vi "Filter Axis Spikes.vi"(8 "Error In":errorcluster, 9 "Axis Enum":T1=enum."Z-axis", 11 "Current Reading":dbl) -> (0 "Error Out":errorcluster, 1 "Axis Enum out":T1=enum."Z-axis", 3 "Filtered Reading":dbl, 5 "Peak Detected?":bool)   [LabVIEW 2013]
doc: "This sub-VI detects peaks due to noise in the positions read by axis encoders and replaces these peaks with\nthe previous value of the axis position."
uses:
  Controls/table_axis_enum.ctl
  <vilib>/ptbypt/NI_PtbyPt.lvlib
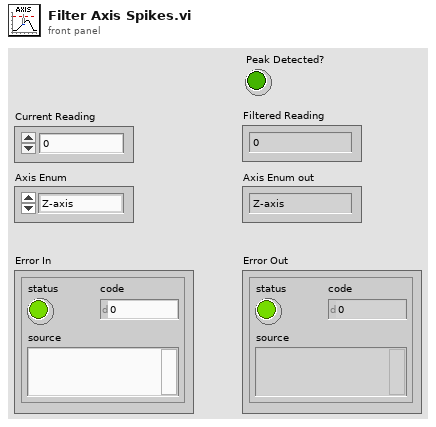
[diagram p1: front panel]
types:
  T1 = typedef "table_axis_enum.ctl" = enum16{"X-axis", "Y-axis", "Z-axis", "W-axis"}
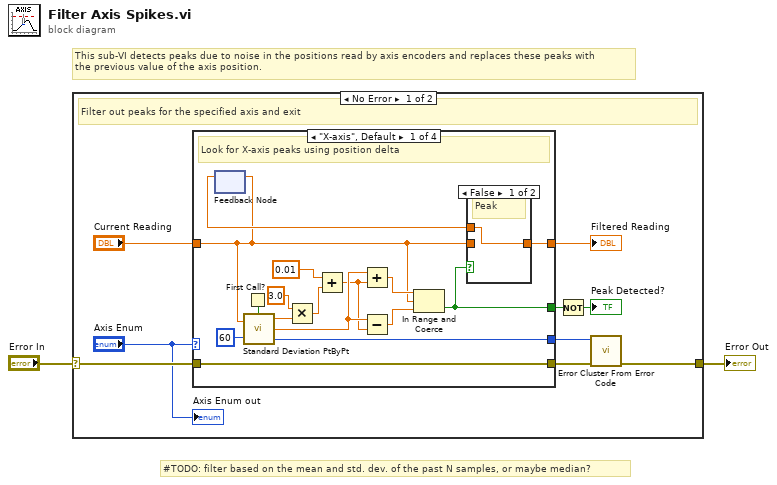
[diagram p0: block diagram]
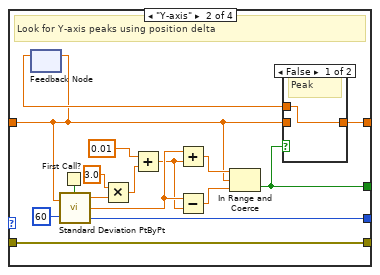
[diagram p3: hidden frame]
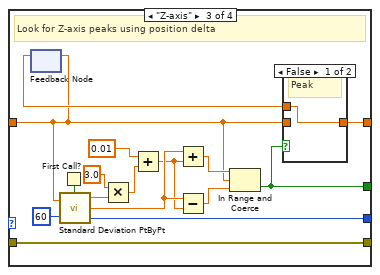
[diagram p5: hidden frame]
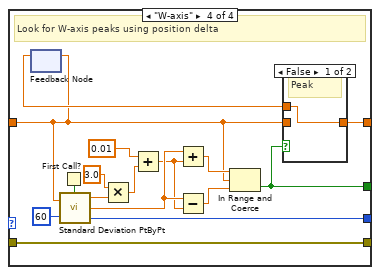
[diagram p7: hidden frame]
diagram:
  # "#TODO: filter based on the mean and std. dev. of the past N samples, or maybe median?"
  # "This sub-VI detects peaks due to noise in the positions read by axis encoders and replaces these peaks with\nthe previous value of the axis position."
  n1 = case shown="No Error" "Error In" {
    selector: "Error In" -> [w11 w84]
    tunnel: [w5 w84] -> w1
    frame No Error {
      # "Filter out peaks for the specified axis and exit"
      n2 = case shown="\"X-axis\", Default" "Axis Enum" {
        tunnel: w11 -> [w27 w45 w63 w81]
        tunnel: [w27 w45 w63 w81] -> w6
        tunnel: "Current Reading" -> [w15 w33 w51 w69]
        tunnel: [w16 w34 w52 w70] -> w9
        tunnel: [w20 w38 w56 w74] -> w8
        tunnel: [w22 w40 w58 w76] -> w4
        frame "X-axis", Default {
          # "Look for X-axis peaks using position delta"
          n3 = feedback-in #1(w15) -> ()
          n4 = feedback #1() -> (w21:dbl)  [unwired: 1 in]
          n5 = First Call?() -> (First Call?: T/F=w26:bool)
          n6 = call <vilib>:"Standard Deviation PtByPt.vi"("x"=w15, "sample length"=60, "initialize"=w26) -> ("standard deviation"=w24:dbl, "mean"=w17:dbl, "error"=w22:i32)
          n7 = Multiply(x=3.0, y=w24) -> (x*y=w14:dbl)
          n8 = Add(x=0.01, y=w14) -> (x+y=w13:dbl)
          n9 = Add(x=w17, y=w13) -> (x+y=w18:dbl)
          n10 = Subtract(x=w17, y=w13) -> (x-y=w19:dbl)
          n11 = In Range and Coerce(upper limit=w18, x=w15, lower limit=w19) -> (In Range?=w16:bool)  [unwired: 1 out]
          n12 = case shown="False" w16 {
            tunnel: w15 -> [_ w29]
            tunnel: w21 -> [w28 _]
            tunnel: [w28 w29] -> w20
            frame False {
              # "Peak"
            }
            frame True {
              # "No peak"
            }
          }
        }
        frame "Y-axis" {
          # "Look for Y-axis peaks using position delta"
          n13 = feedback-in #2(w33) -> ()
          n14 = feedback #2() -> (w39:dbl)  [unwired: 1 in]
          n15 = First Call?() -> (First Call?: T/F=w44:bool)
          n16 = call <vilib>:"Standard Deviation PtByPt.vi"("x"=w33, "sample length"=60, "initialize"=w44) -> ("standard deviation"=w42:dbl, "mean"=w35:dbl, "error"=w40:i32)
          n17 = Multiply(x=3.0, y=w42) -> (x*y=w32:dbl)
          n18 = Add(x=0.01, y=w32) -> (x+y=w31:dbl)
          n19 = Add(x=w35, y=w31) -> (x+y=w36:dbl)
          n20 = Subtract(x=w35, y=w31) -> (x-y=w37:dbl)
          n21 = In Range and Coerce(upper limit=w36, x=w33, lower limit=w37) -> (In Range?=w34:bool)  [unwired: 1 out]
          n22 = case shown="False" w34 {
            tunnel: w33 -> [_ w47]
            tunnel: w39 -> [w46 _]
            tunnel: [w46 w47] -> w38
            frame False {
              # "Peak"
            }
            frame True {
              # "No peak"
            }
          }
        }
        frame "Z-axis" {
          # "Look for Z-axis peaks using position delta"
          n23 = feedback-in #3(w51) -> ()
          n24 = feedback #3() -> (w57:dbl)  [unwired: 1 in]
          n25 = First Call?() -> (First Call?: T/F=w62:bool)
          n26 = call <vilib>:"Standard Deviation PtByPt.vi"("x"=w51, "sample length"=60, "initialize"=w62) -> ("standard deviation"=w60:dbl, "mean"=w53:dbl, "error"=w58:i32)
          n27 = Multiply(x=3.0, y=w60) -> (x*y=w50:dbl)
          n28 = Add(x=0.01, y=w50) -> (x+y=w49:dbl)
          n29 = Add(x=w53, y=w49) -> (x+y=w54:dbl)
          n30 = Subtract(x=w53, y=w49) -> (x-y=w55:dbl)
          n31 = In Range and Coerce(upper limit=w54, x=w51, lower limit=w55) -> (In Range?=w52:bool)  [unwired: 1 out]
          n32 = case shown="False" w52 {
            tunnel: w51 -> [_ w65]
            tunnel: w57 -> [w64 _]
            tunnel: [w64 w65] -> w56
            frame False {
              # "Peak"
            }
            frame True {
              # "No peak"
            }
          }
        }
        frame "W-axis" {
          # "Look for W-axis peaks using position delta"
          n33 = feedback-in #4(w69) -> ()
          n34 = feedback #4() -> (w75:dbl)  [unwired: 1 in]
          n35 = First Call?() -> (First Call?: T/F=w80:bool)
          n36 = call <vilib>:"Standard Deviation PtByPt.vi"("x"=w69, "sample length"=60, "initialize"=w80) -> ("standard deviation"=w78:dbl, "mean"=w71:dbl, "error"=w76:i32)
          n37 = Multiply(x=3.0, y=w78) -> (x*y=w68:dbl)
          n38 = Add(x=0.01, y=w68) -> (x+y=w67:dbl)
          n39 = Add(x=w71, y=w67) -> (x+y=w72:dbl)
          n40 = Subtract(x=w71, y=w67) -> (x-y=w73:dbl)
          n41 = In Range and Coerce(upper limit=w72, x=w69, lower limit=w73) -> (In Range?=w70:bool)  [unwired: 1 out]
          n42 = case shown="False" w70 {
            tunnel: w69 -> [_ w83]
            tunnel: w75 -> [w82 _]
            tunnel: [w82 w83] -> w74
            frame False {
              # "Peak"
            }
            frame True {
              # "No peak"
            }
          }
        }
      }
      "Filtered Reading" <- w8
      n43 = Not(x=w9) -> (.not. x?=→"Peak Detected?":bool)
      n44 = call <vilib>:"Error Cluster From Error Code.vi"("error in (no error)"=w6, "error code (0)"=w4) -> ("error out"=w5:errorcluster)  [unwired: 7 in]
      "Axis Enum out" <- "Axis Enum"
    }
    frame Error {
      # "Pass through and exit"
    }
  }
  "Error Out" <- w1
